vi "FPGA.vi"() -> ()   [LabVIEW 2013]
uses:
  <vilib>/rvi/Emulation/niFpgaSctlEmulationGetInTimedLoop.vi
  <vilib>/rvi/Emulation/niFpgaEmulationReportErrorSimple.vi
  <vilib>/rvi/eio/common/nirviEmuTemplateMethod_errors.vi
  <vilib>/rvi/Emulation/niFpgaGetClockAttributes.vi
  <vilib>/rvi/Emulation/niFpgaCriticalErrorInLSC.vi
  <vilib>/eio/EIONode/EIONode.xnode
panel:
  in  "Watchdog_Kick":bool
  out "Test1":bool
  out "Test2":bool
  out "Test3":bool
  out "Test4":bool
  out "GbxEnc1":i64
  out "GbxEnc2":i64
  out "GbxEnc3":i64
  out "GbxEnc4":i64
  in  "FPGA LED":bool
  out "Chasis Temp":i16
  in  "Motor5":u16=255 max=512 step=1
  in  "Motor6":u16=255 max=512 step=1
  in  "Motor7":u16=255 max=512 step=1
  in  "Motor8":u16=255 max=512 step=1
  in  "Motor9":u16=255 max=512 step=1
  in  "Motor10":u16=255 max=512 step=1
  in  "Motor11":u16=255 max=512 step=1
  in  "Motor12":u16=255 max=512 step=1
  in  "Motor1":u16=255 max=512 step=1
  in  "Motor2":u16=255 max=512 step=1
  in  "Motor3":u16=255 max=512 step=1
  in  "Motor4":u16=255 max=512 step=1
  in  "Halt Execution":bool
  in  "Dout 1":bool
  in  "Dout 2":bool
  in  "Dout 3":bool
  in  "Dout 4":bool
  in  "Dout 5":bool
  in  "Dout 6":bool
  in  "Dout 7":bool
  in  "Dout 8":bool
  out "Din 1":bool
  out "Din 2":bool
  out "Din 3":bool
  out "Din 4":bool
  out "Din 5":bool
  out "Din 6":bool
  out "Din 7":bool
  out "Din 8":bool
  out "Encoder1":i64
  out "Encoder2":i64
  out "Encoder3":i64
  out "Encoder4":i64
  in  "Reset 1":bool
  in  "Reset 2":bool
  in  "Reset 3":bool
  in  "Reset 4":bool
  in  "Analog 2":fxp<+/-,12,5>
  in  "Analog 4":fxp<+/-,12,5>
  in  "Analog 1":fxp<+/-,12,5>
  in  "Analog 3":fxp<+/-,12,5>
  out "PWM counter":i16
  in  "Stop All Motors":bool
  in  "Status LED":bool
  in  "Emergency Stop":bool
  out "Enc1C":bool
  out "Enc2C":bool
  out "Enc3C":bool
  out "Enc4C":bool
  in  "Cal.1":bool
  in  "Cal.2":bool
  in  "Cal. 3":bool
  in  "Cal. 4":bool
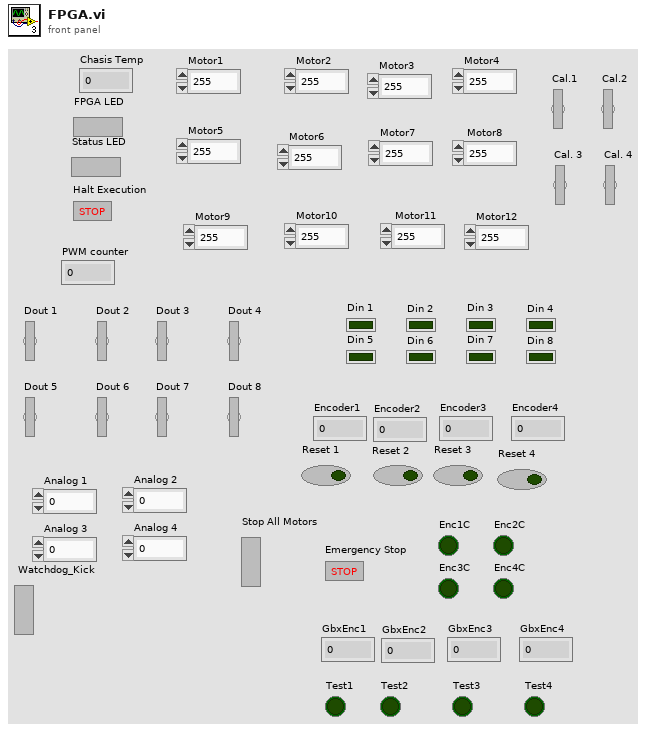
[diagram p1: front panel]
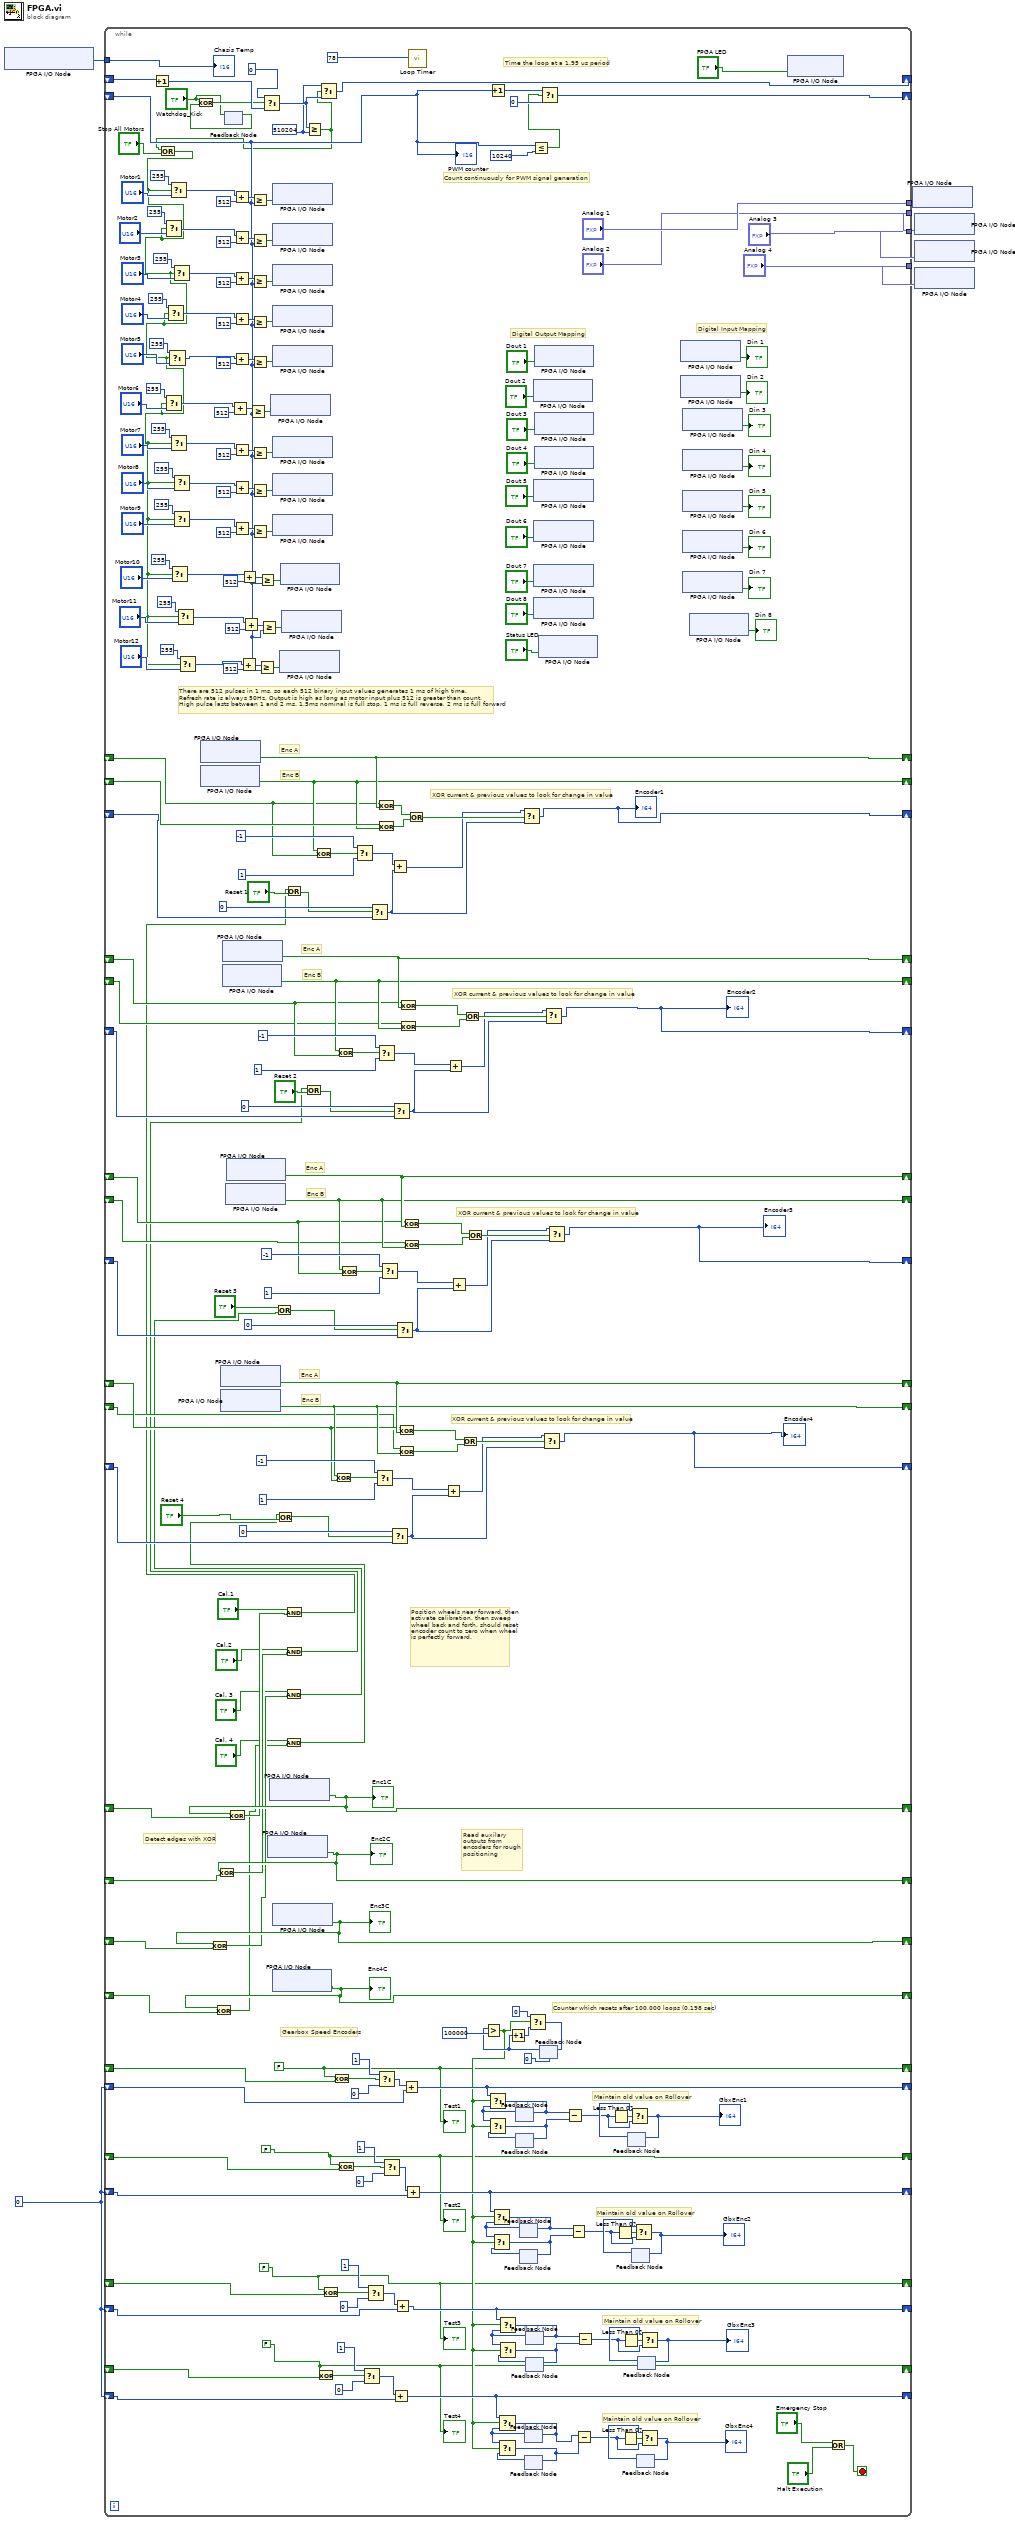
[diagram p0: block diagram]
diagram:
  w1 = u32 0
  n1 = xnode "FPGA I/O Node"() -> ("Chassis Temperature"=w6:i16)  [unwired: 1 in, 1 out]
  n2 = while {
    shift-right: [w234] -> _
    shift-left: _ -> [w218]
    shift-right: [w219] -> _
    shift-left: _ -> [w226]
    shift-right: [w228] -> _
    shift-left: _ -> [w227]
    shift-right: [w206] -> _
    shift-left: _ -> [w204]
    shift-right: [w205] -> _
    shift-left: _ -> [w203]
    shift-right: [w202] -> _
    shift-left: _ -> [w201]
    shift-right: [w190] -> _
    shift-left: _ -> [w188]
    shift-right: [w189] -> _
    shift-left: _ -> [w187]
    shift-right: [w185] -> _
    shift-left: _ -> [w186]
    shift-right: [w173] -> _
    shift-left: _ -> [w170]
    shift-right: [w172] -> _
    shift-left: _ -> [w169]
    shift-right: [w171] -> _
    shift-left: _ -> [w168]
    shift-right: [w163] -> _
    shift-left: _ -> [w162]
    tunnel: w6 -> [w160]
    tunnel: ["Analog 1"] -> w5
    tunnel: ["Analog 2"] -> w4
    tunnel: ["Analog 3"] -> w3
    tunnel: ["Analog 4"] -> w2
    shift-right: [w114] -> _
    shift-left: _ -> [w113]
    shift-right: [w112] -> _
    shift-left: _ -> [w111]
    shift-right: [w110] -> _
    shift-left: _ -> [w109]
    shift-right: [w107] -> _
    shift-left: _ -> [w108]
    shift-right: [w22] -> _
    shift-left: _ -> [w89]
    shift-right: [w21] -> _
    shift-left: _ -> [w76]
    shift-right: [w20] -> _
    shift-left: _ -> [w75]
    shift-right: [w19] -> _
    shift-left: _ -> [w74]
    shift-right: [w60] -> _
    shift-left: w1 -> [w69]
    shift-right: [w37] -> _
    shift-left: w1 -> [w68]
    shift-right: [w36] -> _
    shift-left: w1 -> [w67]
    shift-right: [w32] -> _
    shift-left: w1 -> [w66]
    shift-right: [w17] -> _
    shift-left: _ -> [w18]
    stop <- w117 stop-if-true
    w15 = u32 510204
    w19 = FALSE
    w20 = FALSE
    w21 = FALSE
    w22 = FALSE
    # "Maintain old value on Rollover"
    # "Maintain old value on Rollover"
    # "Maintain old value on Rollover"
    # "Maintain old value on Rollover"
    # "Counter which resets after 100,000 loops (0.198 sec)"
    # "Gearbox Speed Encoders"
    # "Position wheels near forward, then activate calibration, then sweep wheel back and forth. should reset encoder count to zero when wheel is perfectly forward."
    # "Detect edges with XOR"
    # "Read auxilary outputs from encoders for rough positioning"
    # "Count continuously for PWM signal generation"
    # "Time the loop at a 1.95 us period"
    # "XOR current & previous values to look for change in value"
    # "Enc B"
    # "Enc A"
    # "XOR current & previous values to look for change in value"
    # "Enc B"
    # "Enc A"
    # "XOR current & previous values to look for change in value"
    # "Enc B"
    # "Enc A"
    # "XOR current & previous values to look for change in value"
    # "Enc B"
    # "Enc A"
    # "Digital Input Mapping"
    # "Digital Output Mapping"
    # "There are 512 pulses in 1 ms, so each 512 binary input values generates 1 ms of high time.\nRefresh rate is always 50Hz. Output is high as long as motor input plus 512 is greater than count.\nHigh pulse lasts between 1 and 2 ms. 1.5ms nominal is full stop, 1 ms is full reverse, 2 ms is full forward"
    n3 = Increment(x=w18) -> (x+1=w11:u32)
    n4 = xnode "FPGA I/O Node"() -> ("Port7/DIO1"=w219:bool)  [unwired: 1 in, 1 out]
    n5 = xnode "FPGA I/O Node"() -> ("Port7/DIO0"=w234:bool)  [unwired: 1 in, 1 out]
    n6 = xnode "FPGA I/O Node"() -> ("Port4/DIO1"=w172:bool)  [unwired: 1 in, 1 out]
    n7 = xnode "FPGA I/O Node"() -> ("Port4/DIO0"=w173:bool)  [unwired: 1 in, 1 out]
    n8 = xnode "FPGA I/O Node"() -> ("Port3/DIO1"=w205:bool)  [unwired: 1 in, 1 out]
    n9 = xnode "FPGA I/O Node"() -> ("Port3/DIO0"=w206:bool)  [unwired: 1 in, 1 out]
    n10 = feedback-in #1("Watchdog_Kick") -> ()
    n11 = feedback #1() -> (w8:bool)  [unwired: 1 in]
    n12 = Exclusive Or(1:w8, 2:"Watchdog_Kick") -> (0:w9:bool)
    n13 = xnode "FPGA I/O Node"() -> ("Port3/DIO6"=w189:bool)  [unwired: 1 in, 1 out]
    n14 = xnode "FPGA I/O Node"() -> ("Port3/DIO5"=w190:bool)  [unwired: 1 in, 1 out]
    n15 = Select(t=u32 0, s=w9, f=w11) -> (s? t:f=w16:u32)
    n16 = xnode "FPGA I/O Node"() -> ("Port3/DIO2"=w112:bool)  [unwired: 1 in, 1 out]
    "Enc2C" <- w112
    n17 = Exclusive Or(1:w111, 2:w112) -> (0:w105:bool)
    n18 = xnode "FPGA I/O Node"() -> ("Port7/DIO2"=w114:bool)  [unwired: 1 in, 1 out]
    "Enc1C" <- w114
    n19 = Exclusive Or(1:w113, 2:w114) -> (0:w106:bool)
    n20 = xnode "FPGA I/O Node"() -> ("Port4/DIO2"=w107:bool)  [unwired: 1 in, 1 out]
    "Enc4C" <- w107
    n21 = Exclusive Or(1:w108, 2:w107) -> (0:w103:bool)
    n22 = xnode "FPGA I/O Node"() -> ("Port3/DIO7"=w110:bool)  [unwired: 1 in, 1 out]
    "Enc3C" <- w110
    n23 = Exclusive Or(1:w109, 2:w110) -> (0:w104:bool)
    n24 = And(x="Cal. 3", y=w104) -> (x .and. y?=w91:bool)
    n25 = Or(x="Reset 3", y=w91) -> (x .or. y?=w96:bool)
    n26 = And(x="Cal. 4", y=w103) -> (x .and. y?=w90:bool)
    n27 = Or(x=w90, y="Reset 4") -> (x .or. y?=w97:bool)
    n28 = And(x="Cal.1", y=w106) -> (x .and. y?=w93:bool)
    n29 = Or(x=w93, y="Reset 1") -> (x .or. y?=w94:bool)
    n30 = And(x="Cal.2", y=w105) -> (x .and. y?=w92:bool)
    n31 = Or(x=w92, y="Reset 2") -> (x .or. y?=w95:bool)
    n32 = Greater Or Equal?(x=w16, y=w15) -> (x >= y?=w12:bool)
    n33 = Or(x=w12, y="Stop All Motors") -> (x .or. y?=w14:bool)
    n34 = Select(t=i16 255, s=w14, f="Motor2") -> (s? t:f=w140:u16)
    n35 = Select(t=i16 255, s=w14, f="Motor6") -> (s? t:f=w132:u16)
    n36 = Select(t=i16 255, s=w14, f="Motor4") -> (s? t:f=w136:u16)
    n37 = Select(t=i16 255, s=w14, f="Motor5") -> (s? t:f=w134:u16)
    n38 = Select(t=i16 255, s=w14, f="Motor1") -> (s? t:f=w142:u16)
    n39 = Select(t=i16 255, s=w14, f="Motor7") -> (s? t:f=w130:u16)
    n40 = Select(t=i16 255, s=w14, f="Motor10") -> (s? t:f=w124:u16)
    n41 = Select(t=i16 255, s=w14, f="Motor3") -> (s? t:f=w138:u16)
    n42 = Select(t=i16 255, s=w14, f="Motor8") -> (s? t:f=w128:u16)
    n43 = Select(t=i16 255, s=w14, f="Motor9") -> (s? t:f=w126:u16)
    n44 = Select(t=i16 255, s=w14, f="Motor11") -> (s? t:f=w122:u16)
    n45 = Select(t=i16 255, s=w14, f="Motor12") -> (s? t:f=w120:u16)
    n46 = Add(x=w132, y=i16 512) -> (x+y=w276:u16)
    n47 = Add(x=w142, y=i16 512) -> (x+y=w286:u16)
    n48 = Add(x=w140, y=i16 512) -> (x+y=w284:u16)
    n49 = Add(x=w138, y=i16 512) -> (x+y=w282:u16)
    n50 = Add(x=w136, y=i16 512) -> (x+y=w280:u16)
    n51 = Add(x=w134, y=i16 512) -> (x+y=w278:u16)
    n52 = Add(x=w130, y=i16 512) -> (x+y=w274:u16)
    n53 = Add(x=w128, y=i16 512) -> (x+y=w272:u16)
    n54 = Add(x=w126, y=i16 512) -> (x+y=w270:u16)
    n55 = Add(x=w120, y=i16 512) -> (x+y=w264:u16)
    n56 = Add(x=w124, y=i16 512) -> (x+y=w268:u16)
    n57 = Add(x=w122, y=i16 512) -> (x+y=w266:u16)
    n58 = Greater Or Equal?(x=w276, y=w162) -> (x >= y?=w257:bool)
    n59 = Greater Or Equal?(x=w286, y=w162) -> (x >= y?=w262:bool)
    n60 = Greater Or Equal?(x=w284, y=w162) -> (x >= y?=w261:bool)
    n61 = Greater Or Equal?(x=w282, y=w162) -> (x >= y?=w260:bool)
    n62 = Greater Or Equal?(x=w280, y=w162) -> (x >= y?=w259:bool)
    n63 = Greater Or Equal?(x=w278, y=w162) -> (x >= y?=w258:bool)
    n64 = Greater Or Equal?(x=w274, y=w162) -> (x >= y?=w256:bool)
    n65 = Greater Or Equal?(x=w272, y=w162) -> (x >= y?=w255:bool)
    n66 = Greater Or Equal?(x=w270, y=w162) -> (x >= y?=w254:bool)
    n67 = Greater Or Equal?(x=w264, y=w162) -> (x >= y?=w251:bool)
    n68 = Greater Or Equal?(x=w268, y=w162) -> (x >= y?=w253:bool)
    n69 = Greater Or Equal?(x=w266, y=w162) -> (x >= y?=w252:bool)
    n70 = xnode "FPGA I/O Node"("Port0/DIO5"=w257) -> ()  [unwired: 1 in, 1 out]
    n71 = xnode "FPGA I/O Node"("Port0/DIO0"=w262) -> ()  [unwired: 1 in, 1 out]
    n72 = xnode "FPGA I/O Node"("Port0/DIO1"=w261) -> ()  [unwired: 1 in, 1 out]
    n73 = xnode "FPGA I/O Node"("Port0/DIO2"=w260) -> ()  [unwired: 1 in, 1 out]
    n74 = xnode "FPGA I/O Node"("Port0/DIO3"=w259) -> ()  [unwired: 1 in, 1 out]
    n75 = xnode "FPGA I/O Node"("Port0/DIO4"=w258) -> ()  [unwired: 1 in, 1 out]
    n76 = xnode "FPGA I/O Node"("Port0/DIO6"=w256) -> ()  [unwired: 1 in, 1 out]
    n77 = xnode "FPGA I/O Node"("Port0/DIO7"=w255) -> ()  [unwired: 1 in, 1 out]
    n78 = xnode "FPGA I/O Node"("Port0/DIO8"=w254) -> ()  [unwired: 1 in, 1 out]
    n79 = xnode "FPGA I/O Node"("Port9/DIO4"=w251) -> ()  [unwired: 1 in, 1 out]
    n80 = xnode "FPGA I/O Node"("Port1/DIO9"=w253) -> ()  [unwired: 1 in, 1 out]
    n81 = xnode "FPGA I/O Node"("Port9/DIO6"=w252) -> ()  [unwired: 1 in, 1 out]
    n82 = Exclusive Or(1:w218, 2:w219) -> (0:w220:bool)
    n83 = Exclusive Or(1:w74, 2:w19) -> (0:w77:bool)
    n84 = Select(t=w15, s=w12, f=w16) -> (s? t:f=w17:u32)
    n85 = Exclusive Or(1:w75, 2:w20) -> (0:w80:bool)
    n86 = Exclusive Or(1:w89, 2:w22) -> (0:w86:bool)
    n87 = Exclusive Or(1:w170, 2:w172) -> (0:w174:bool)
    n88 = Exclusive Or(1:w204, 2:w205) -> (0:w208:bool)
    n89 = Exclusive Or(1:w76, 2:w21) -> (0:w83:bool)
    n90 = Exclusive Or(1:w188, 2:w189) -> (0:w191:bool)
    n91 = Select(t=i16 -1, s=w220, f=i16 1) -> (s? t:f=w222:i16)
    n92 = Select(t=i16 1, s=w77, f=i16 0) -> (s? t:f=w70:i16)
    n93 = Select(t=i16 1, s=w80, f=i16 0) -> (s? t:f=w71:i16)
    n94 = Select(t=i16 0, s=w94, f=w227) -> (s? t:f=w223:i16)
    n95 = Select(t=i16 -1, s=w174, f=i16 1) -> (s? t:f=w176:i16)
    n96 = Exclusive Or(1:w234, 2:w218) -> (0:w233:bool)
    n97 = Exclusive Or(1:w219, 2:w226) -> (0:w232:bool)
    n98 = Select(t=i16 -1, s=w208, f=i16 1) -> (s? t:f=w210:i16)
    n99 = Select(t=i16 1, s=w86, f=i16 0) -> (s? t:f=w73:i16)
    n100 = Select(t=i16 -1, s=w191, f=i16 1) -> (s? t:f=w193:i16)
    n101 = Select(t=i16 1, s=w83, f=i16 0) -> (s? t:f=w72:i16)
    n102 = Add(x=w222, y=w223) -> (x+y=w221:i16)
    n103 = Select(t=i16 0, s=w97, f=w168) -> (s? t:f=w177:i16)
    n104 = Add(x=w70, y=w66) -> (x+y=w32:u32)
    n105 = Select(t=i16 0, s=w95, f=w201) -> (s? t:f=w211:i16)
    n106 = Add(x=w71, y=w67) -> (x+y=w36:u32)
    n107 = Select(t=i16 0, s=w96, f=w186) -> (s? t:f=w194:i16)
    n108 = Exclusive Or(1:w173, 2:w170) -> (0:w183:bool)
    n109 = Exclusive Or(1:w172, 2:w169) -> (0:w182:bool)
    n110 = Exclusive Or(1:w206, 2:w204) -> (0:w217:bool)
    n111 = Exclusive Or(1:w205, 2:w203) -> (0:w216:bool)
    n112 = Add(x=w73, y=w69) -> (x+y=w60:u32)
    n113 = Exclusive Or(1:w190, 2:w188) -> (0:w200:bool)
    n114 = Exclusive Or(1:w189, 2:w187) -> (0:w199:bool)
    n115 = Add(x=w72, y=w68) -> (x+y=w37:u32)
    n116 = Or(x=w233, y=w232) -> (x .or. y?=w231:bool)
    n117 = call "Loop Timer"("Count(Ticks)"=i16 78) -> ()  [unwired: 1 out]
    n118 = Add(x=w176, y=w177) -> (x+y=w175:i16)
    n119 = Add(x=w210, y=w211) -> (x+y=w209:i16)
    n120 = Add(x=w193, y=w194) -> (x+y=w192:i16)
    n121 = Or(x=w183, y=w182) -> (x .or. y?=w181:bool)
    n122 = Or(x=w217, y=w216) -> (x .or. y?=w215:bool)
    n123 = Or(x=w200, y=w199) -> (x .or. y?=w198:bool)
    n124 = Increment(x=w162) -> (x+1=w167:i16)
    n125 = feedback #2() -> (w59:u32)  [unwired: 1 in]
    n126 = feedback #3() -> (w58:u32)  [unwired: 1 in]
    n127 = feedback #4() -> (w52:u32)  [unwired: 1 in]
    n128 = feedback #5() -> (w51:u32)  [unwired: 1 in]
    n129 = Select(t=w221, s=w231, f=w223) -> (s? t:f=w228:i16)
    "Encoder1" <- w228
    n130 = feedback #6() -> (w42:u32)  [unwired: 1 in]
    n131 = feedback #7() -> (w41:u32)  [unwired: 1 in]
    n132 = feedback #8() -> (w47:u32)  [unwired: 1 in]
    n133 = feedback #9() -> (w46:u32)  [unwired: 1 in]
    n134 = Less Or Equal?(x=w162, y=i16 10240) -> (x <= y?=w165:bool)
    n135 = xnode "FPGA I/O Node"("Port1/DIO3"="Dout 2") -> ()  [unwired: 1 in, 1 out]
    n136 = xnode "FPGA I/O Node"("Port1/DIO6"="Dout 5") -> ()  [unwired: 1 in, 1 out]
    n137 = xnode "FPGA I/O Node"("Port1/DIO7"="Dout 6") -> ()  [unwired: 1 in, 1 out]
    n138 = xnode "FPGA I/O Node"("Port1/DIO8"="Dout 7") -> ()  [unwired: 1 in, 1 out]
    n139 = xnode "FPGA I/O Node"("Port2/DIO9"="Dout 8") -> ()  [unwired: 1 in, 1 out]
    n140 = xnode "FPGA I/O Node"("Port1/DIO2"="Dout 1") -> ()  [unwired: 1 in, 1 out]
    n141 = xnode "FPGA I/O Node"("Port1/DIO4"="Dout 3") -> ()  [unwired: 1 in, 1 out]
    n142 = xnode "FPGA I/O Node"("Port1/DIO5"="Dout 4") -> ()  [unwired: 1 in, 1 out]
    n143 = xnode "FPGA I/O Node"("Port2/DIO1"="Status LED") -> ()  [unwired: 1 in, 1 out]
    n144 = feedback #10(u32 0) -> (w63:u32)
    n145 = Greater?(x=w63, y=u32 100000) -> (0:w31:bool)
    n146 = Select(t=w60, s=w31, f=w59) -> (s? t:f=w24:u32)
    n147 = Select(t=w59, s=w31, f=w58) -> (s? t:f=w23:u32)
    n148 = Select(t=w37, s=w31, f=w52) -> (s? t:f=w26:u32)
    n149 = Select(t=w52, s=w31, f=w51) -> (s? t:f=w25:u32)
    n150 = Select(t=w32, s=w31, f=w42) -> (s? t:f=w30:u32)
    n151 = Select(t=w42, s=w31, f=w41) -> (s? t:f=w29:u32)
    n152 = Select(t=w36, s=w31, f=w47) -> (s? t:f=w28:u32)
    n153 = Select(t=w47, s=w31, f=w46) -> (s? t:f=w27:u32)
    n154 = Increment(x=w63) -> (x+1=w64:u32)
    n155 = feedback-in #2(w24) -> ()
    n156 = feedback-in #3(w23) -> ()
    n157 = feedback-in #4(w26) -> ()
    n158 = feedback-in #5(w25) -> ()
    n159 = feedback-in #6(w30) -> ()
    n160 = feedback-in #7(w29) -> ()
    n161 = feedback-in #8(w28) -> ()
    n162 = feedback-in #9(w27) -> ()
    n163 = Select(t=u32 0, s=w31, f=w64) -> (s? t:f=w62:u32)
    n164 = feedback-in #10(w62) -> ()
    n165 = Select(t=w167, s=w165, f=i16 0) -> (s? t:f=w163:i16)
    n166 = Select(t=w175, s=w181, f=w177) -> (s? t:f=w171:i16)
    "Encoder4" <- w171
    n167 = Select(t=w209, s=w215, f=w211) -> (s? t:f=w202:i16)
    "Encoder2" <- w202
    n168 = Select(t=w192, s=w198, f=w194) -> (s? t:f=w185:i16)
    "Encoder3" <- w185
    n169 = Subtract(x=w24, y=w23) -> (x-y=w53:i64)
    n170 = Subtract(x=w26, y=w25) -> (x-y=w48:i64)
    n171 = Subtract(x=w30, y=w29) -> (x-y=w38:i64)
    n172 = Subtract(x=w28, y=w27) -> (x-y=w43:i64)
    n173 = Less Than 0?(x=w53) -> (x < 0?=w56:bool)
    n174 = Less Than 0?(x=w48) -> (x < 0?=w50:bool)
    n175 = Less Than 0?(x=w38) -> (x < 0?=w40:bool)
    n176 = Less Than 0?(x=w43) -> (x < 0?=w45:bool)
    n177 = feedback #11() -> (w54:i64)  [unwired: 1 in]
    n178 = Select(t=w54, s=w56, f=w53) -> (s? t:f=w55:i64)
    "GbxEnc1" <- w55
    n179 = feedback-in #11(w55) -> ()
    n180 = feedback #12() -> (w49:i64)  [unwired: 1 in]
    n181 = Select(t=w49, s=w50, f=w48) -> (s? t:f=w35:i64)
    "GbxEnc2" <- w35
    n182 = feedback-in #12(w35) -> ()
    n183 = feedback #13() -> (w39:i64)  [unwired: 1 in]
    n184 = feedback #14() -> (w44:i64)  [unwired: 1 in]
    n185 = Select(t=w39, s=w40, f=w38) -> (s? t:f=w33:i64)
    "GbxEnc4" <- w33
    n186 = feedback-in #13(w33) -> ()
    n187 = Select(t=w44, s=w45, f=w43) -> (s? t:f=w34:i64)
    "GbxEnc3" <- w34
    n188 = feedback-in #14(w34) -> ()
    n189 = xnode "FPGA I/O Node"() -> ("Port3/DIO8"=→"Din 1":bool)  [unwired: 1 in, 1 out]
    n190 = xnode "FPGA I/O Node"() -> ("Port4/DIO9"=→"Din 2":bool)  [unwired: 1 in, 1 out]
    n191 = xnode "FPGA I/O Node"() -> ("Port4/DIO3"=→"Din 3":bool)  [unwired: 1 in, 1 out]
    n192 = xnode "FPGA I/O Node"() -> ("Port4/DIO4"=→"Din 4":bool)  [unwired: 1 in, 1 out]
    n193 = xnode "FPGA I/O Node"() -> ("Port4/DIO5"=→"Din 5":bool)  [unwired: 1 in, 1 out]
    n194 = xnode "FPGA I/O Node"() -> ("Port4/DIO6"=→"Din 6":bool)  [unwired: 1 in, 1 out]
    n195 = xnode "FPGA I/O Node"() -> ("Port9/DIO2"=→"Din 7":bool)  [unwired: 1 in, 1 out]
    n196 = xnode "FPGA I/O Node"() -> ("Port9/DIO9"=→"Din 8":bool)  [unwired: 1 in, 1 out]
    n197 = xnode "FPGA I/O Node"("FPGA LED"="FPGA LED") -> ()  [unwired: 1 in, 1 out]
    n198 = Or(x="Emergency Stop", y="Halt Execution") -> (x .or. y?=w117:bool)
    "Chasis Temp" <- w160
    "PWM counter" <- w162
    "Test4" <- w19
    "Test3" <- w20
    "Test2" <- w21
    "Test1" <- w22
  }
  n199 = xnode "FPGA I/O Node"("ModB/AO0"=w5) -> ()  [unwired: 1 in, 1 out]
  n200 = xnode "FPGA I/O Node"("ModB/AO1"=w4) -> ()  [unwired: 1 in, 1 out]
  n201 = xnode "FPGA I/O Node"("ModB/AO2"=w3) -> ()  [unwired: 1 in, 1 out]
  n202 = xnode "FPGA I/O Node"("ModB/AO3"=w2) -> ()  [unwired: 1 in, 1 out]
